vi "DeleteActionToBuffer.vi"() -> ()   [LabVIEW 2019]
panel:
  in  "error in (no error)":errorcluster
  in  "Remaining Action":refnum<vi>
  out "error out":errorcluster
  in  "ManualFlg":bool
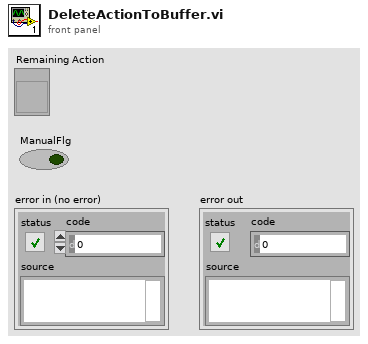
[diagram p1: front panel]
types:
  T1 = enum16{"Initial", "Add", "Read", "Delete & Check"}
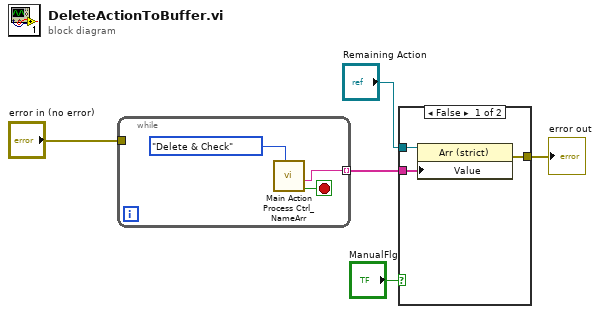
[diagram p0: block diagram]
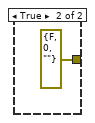
[diagram p2: hidden frame]
diagram:
  n1 = while {
    tunnel: "error in (no error)" -> [_]
    tunnel: [w6] -> w3 mode=indexing
    stop <- w7 stop-if-true
    n2 = call "Main Action Process Ctrl_NameArr.vi"("Action"=T1."Delete & Check") -> ("Finish"=w7:bool, "Delete Action"=w6:string)  [unwired: 6 in, 3 out]
  }
  n3 = case shown="False" "ManualFlg" {
    tunnel: "Remaining Action" -> [w11 _]
    tunnel: w3 -> [w10 _]
    tunnel: [w9 errorcluster {"status"=FALSE, "code"=0, "source"=""} ("error out")] -> w4
    frame False {
      n4 = property class="Arr (strict)"(reference=w11, "Value"=w10) -> (error out=w9:errorcluster)  [unwired: 1 in, 1 out]
    }
    frame True {
    }
  }
  "error out" <- w4
